vi "SetROI.vi"(7 "error in (no error)":errorcluster, 9 "SizeIn":T1, 10 "Handle in":u32) -> (0 "error out":errorcluster, 2 "sizeout":T1, 3 "Handle out":u32)   [LabVIEW 2015]
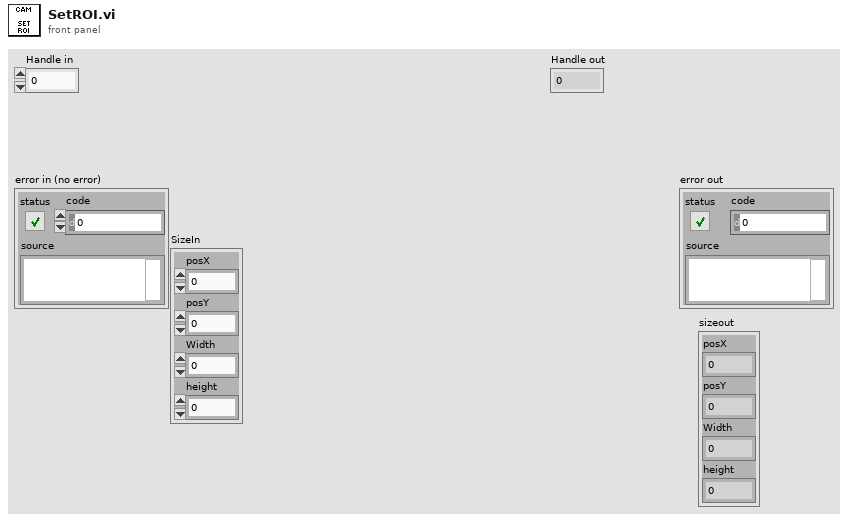
[diagram p1: front panel]
types:
  T1 = cluster{"posX":i32, "posY":i32, "Width":i32, "height":i32}
  T2 = typedef "LVMinMaxIncTypeDef.ctl" = cluster{"Minimum":dbl, "Maximum":dbl, "Increment":dbl}
  T3 = cluster{"H Offset":cluster{"Value":i32, "Limits":T2}, "V Offset":cluster{"Value":i32, "Limits":T2}, "H Size":cluster{"Value":i32, "Limits":T2}, "V Size":cluster{"Value":i32, "Limits":T2}}
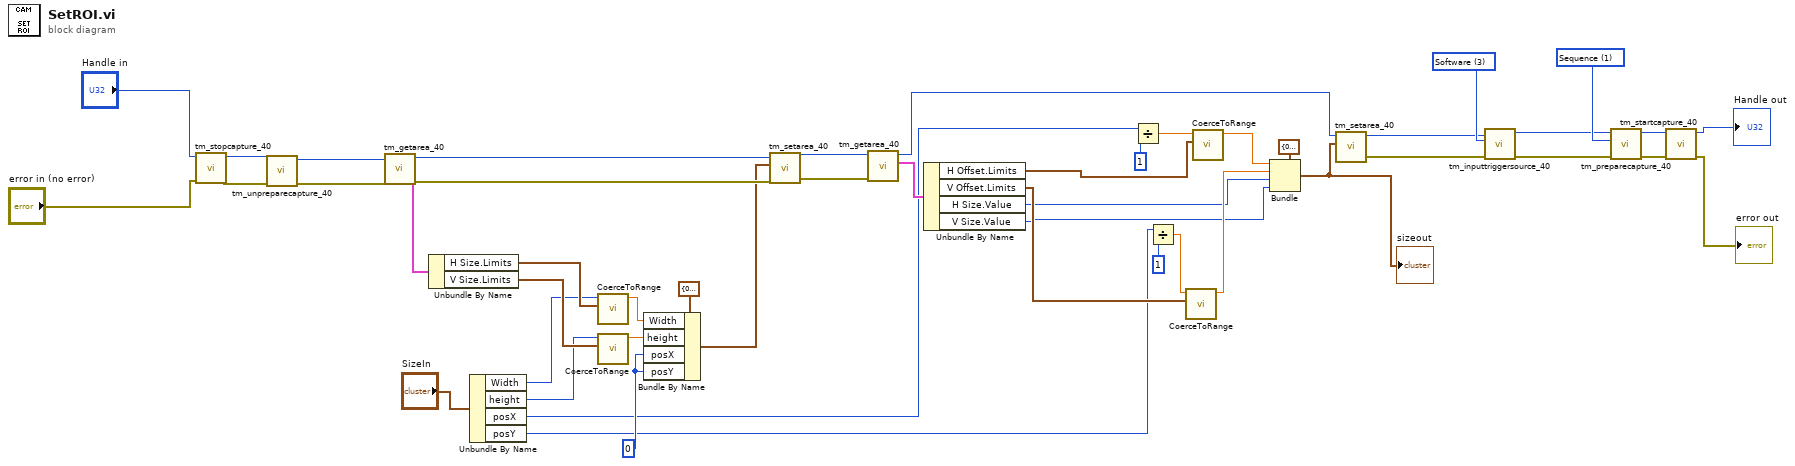
[diagram p0: block diagram]
diagram:
  w15 = 3 items=["Internal"=1, "External"=2, "Software"=3, "Master Pulse"=4] ("Source")
  w16 = 1 items=["Snap", "Sequence"] ("Capture mode")
  w21 = 0 ("posX")
  n1 = call <userlib>:"tm_stopcapture_40.vi"("error in (no error)"="error in (no error)", "Handle in"="Handle in") -> ("error out"=w5:errorcluster, "Handle out"=w6:u32)  [unwired: 8 in]
  n2 = call <userlib>:"tm_unpreparecapture_40.vi"("error in (no error)"=w5, "Handle in"=w6) -> ("error out"=w12:errorcluster, "Handle out"=w11:u32)  [unwired: 8 in]
  n3 = call <userlib>:"tm_getarea_40.vi"("error in (no error)"=w12, "Handle in"=w11) -> ("error out"=w42:errorcluster, "Sub Region"=w43:T3, "Handle out"=w41:u32)  [unwired: 7 in]
  n4 = Unbundle By Name(w43) -> ("H Size.Limits"=w40:T2, "V Size.Limits"=w39:T2)
  n5 = Unbundle By Name("SizeIn") -> ("Width"=w38:i32, "height"=w37:i32, "posX"=w18:i32, "posY"=w17:i32)
  n6 = call "CoerceToRange.vi"("Range"=w40, "input"=w38) -> ("coerced"=w33:dbl)  [unwired: 9 in]
  n7 = call "CoerceToRange.vi"("Range"=w39, "input"=w37) -> ("coerced"=w34:dbl)  [unwired: 9 in]
  n8 = Bundle By Name(cluster=T1 {"posX"=0, "posY"=0, "Width"=0, "height"=0} ("SizeIn"), "Width"=w33, "height"=w34, "posX"=w21, "posY"=w21) -> (w32:T1)
  n9 = call <userlib>:"tm_setarea_40.vi"("error in (no error)"=w42, "Sub Region"=w32, "Handle in"=w41) -> ("error out"=w31:errorcluster, "Handle out"=w30:u32)  [unwired: 7 in]
  n10 = call <userlib>:"tm_getarea_40.vi"("error in (no error)"=w31, "Handle in"=w30) -> ("Sub Region"=w29:T3, "Handle out"=w23:u32)  [unwired: 7 in, 1 out]
  n11 = Unbundle By Name(w29) -> ("H Offset.Limits"=w28:T2, "V Offset.Limits"=w27:T2, "H Size.Value"=w20:i32, "V Size.Value"=w19:i32)
  n12 = Divide(x=w18, y=1) -> (x/y=w46:dbl)
  n13 = Divide(x=w17, y=1) -> (x/y=w44:dbl)
  n14 = call "CoerceToRange.vi"("Range"=w27, "input"=w44) -> ("coerced"=w24:dbl)  [unwired: 9 in]
  n15 = call "CoerceToRange.vi"("Range"=w28, "input"=w46) -> ("coerced"=w25:dbl)  [unwired: 9 in]
  n16 = Bundle(cluster=T1 {"posX"=0, "posY"=0, "Width"=0, "height"=0} ("sizeout"), "posX"=w25, "posY"=w24, "Width"=w20, "height"=w19) -> (w22:T1)
  "sizeout" <- w22
  n17 = call <userlib>:"tm_setarea_40.vi"("Sub Region"=w22, "Handle in"=w23) -> ("error out"=w9:errorcluster, "Handle out"=w10:u32)  [unwired: 8 in]
  n18 = call <userlib>:"tm_inputtriggersource_40.vi"("error in (no error)"=w9, "Source"=w15, "Handle in"=w10) -> ("error out"=w14:errorcluster, "Handle out"=w13:u32)  [unwired: 7 in]
  n19 = call <userlib>:"tm_preparecapture_40.vi"("error in (no error)"=w14, "Capture mode"=w16, "Handle in"=w13) -> ("error out"=w3:errorcluster, "Handle out"=w4:u32)  [unwired: 5 in, 2 out]
  n20 = call <userlib>:"tm_startcapture_40.vi"("error in (no error)"=w3, "Handle in"=w4) -> ("error out"=→"error out":errorcluster, "Handle out"=→"Handle out":u32)  [unwired: 8 in]
